vi "Set Sender.vi"(10 "Sender":refnum<class "Sender.lvclass">, 11 "Last Ack Msg Strategy in":refnum<class "Last Ack Msg Strategy.lvclass">) -> (3 "Last Ack Msg Strategy out":refnum<class "Last Ack Msg Strategy.lvclass">)   [LabVIEW 2021, in "jettl.lvlib" / "Last Ack Msg Strategy.lvlib" / "Last Ack Msg Strategy.lvclass"]
uses:
  Last Ack Msg Strategy.lvclass
  Last Ack Msg Strategy.lvclass/Last Ack Msg Strategy.ctl
  Sender/Sender/Sender.lvclass
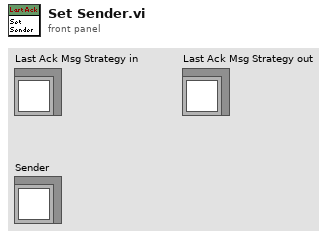
[diagram p1: front panel]
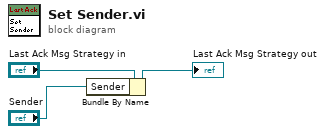
[diagram p0: block diagram]
diagram:
  n1 = Bundle By Name(cluster="Last Ack Msg Strategy in", "Sender"="Sender") -> (→"Last Ack Msg Strategy out":refnum<class "Last Ack Msg Strategy.lvclass">)
